vi "Edycja_kursorow_.vi"(7 "Wykres":waveform(dbl)[](array[waveform]), 8 "error in (no error)":errorcluster, 10 "Zablokowane free in":T1[](array[typedef]), 11 "Wykres Ref":refnum<vi>) -> (0 "error out":errorcluster, 2 "Zablokowane free out":T1[](array[typedef]))   [LabVIEW 2013]
uses:
  Kontrolki/GUI/Edycja_blokowanie_free.ctl
panel:
  in  "(Kursor 2)":i32(ring) caption="Lista przebiegów" items=["Przebieg 0", "Przebieg 1", "Przebieg 2", "Przebieg 3", "Kursor", "\"Swobodny\""]
  in  "(Kursor 1)":i32(ring) caption="Lista przebiegów" items=["Przebieg 0", "Przebieg 1", "Przebieg 2", "Przebieg 3", "Kursor", "\"Swobodny\""]
  in  "Lista aktywnych kursorów":i32(ring) items=["Pom1", "Pom2", "Kur_swob", "Kur_2_3"]
  in  "Cancel Button":bool
  in  "OK Button":bool
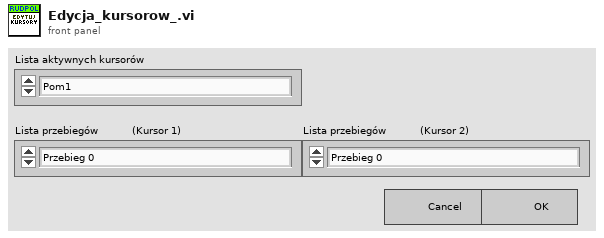
[diagram p1: front panel]
types:
  T1 = typedef "Edycja_blokowanie_free.ctl" = cluster{"Pozycja Y":dbl, "Pozycja X":dbl, "BlokujX":bool, "BlokujY":bool, "Zablokowane":i32}
  T2 = cluster{"Aktywny kursor":i32, "typ kursora":u32, "Aktywne przebiegi":i32[]}
  T3 = typedef "LVCursorListTypeDef.ctl" = cluster{"Name":string, "Color":u32, "Style":u8, "Point Style":u8, "Name Visible":bool, "Allow Drag":bool, "Cursor Mode":u32, "Plot":i32, "Index":i32, "Position":cluster{"X":dbl, "Y":dbl}, "X Scale":u32, "Y Scale":u32, "Watch Plots":i32[], "Watch All Plots":bool, "Plot Area":i32, "Label Offset":cluster{"X":dbl, "Y":dbl}}[]
  T4 = cluster{"Name":string, "Color":u32, "Style":u8, "Point Style":u8, "Name Visible":bool, "Allow Drag":bool, "Cursor Mode":u32, "Plot":i32, "Index":i32, "Position":cluster{"X":dbl, "Y":dbl}, "X Scale":u32, "Y Scale":u32, "Watch Plots":i32[], "Watch All Plots":bool, "Plot Area":i32, "Label Offset":cluster{"X":dbl, "Y":dbl}}
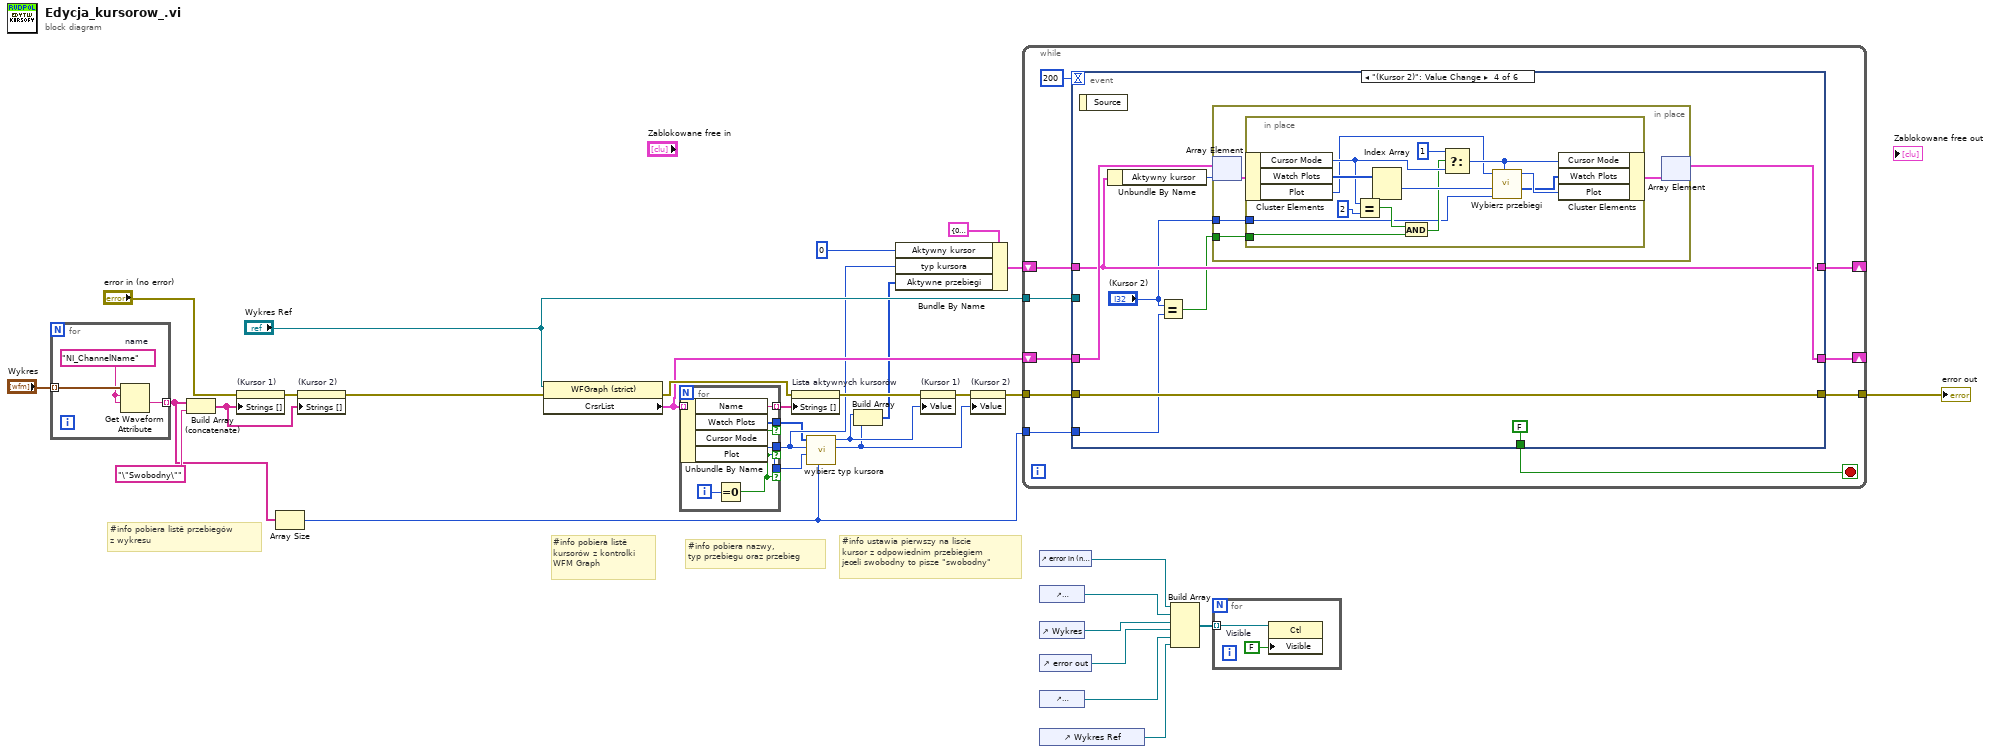
[diagram p0: block diagram]
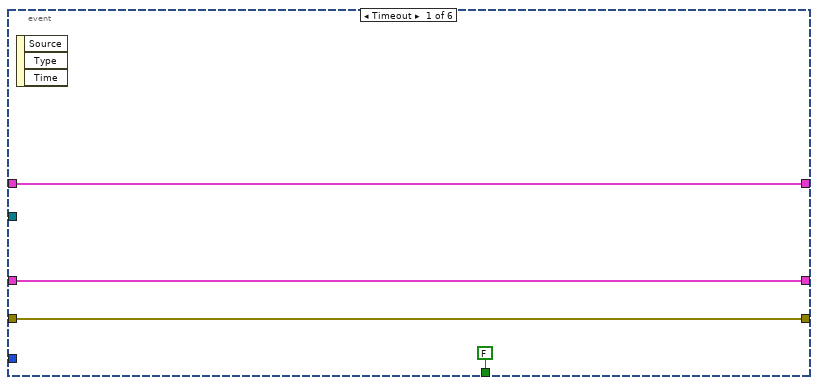
[diagram p2: hidden frame]
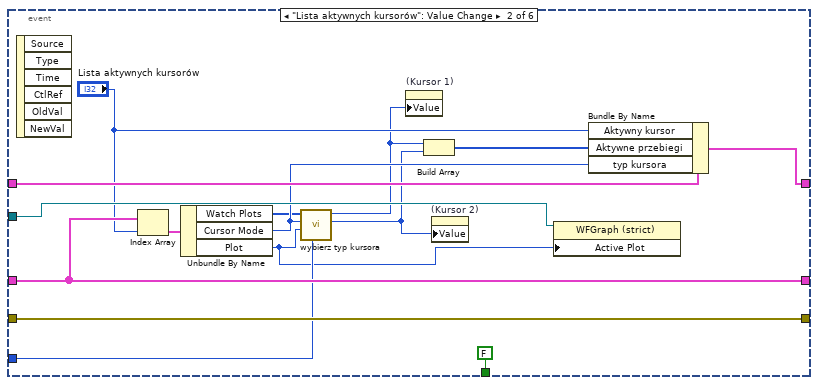
[diagram p3: hidden frame]
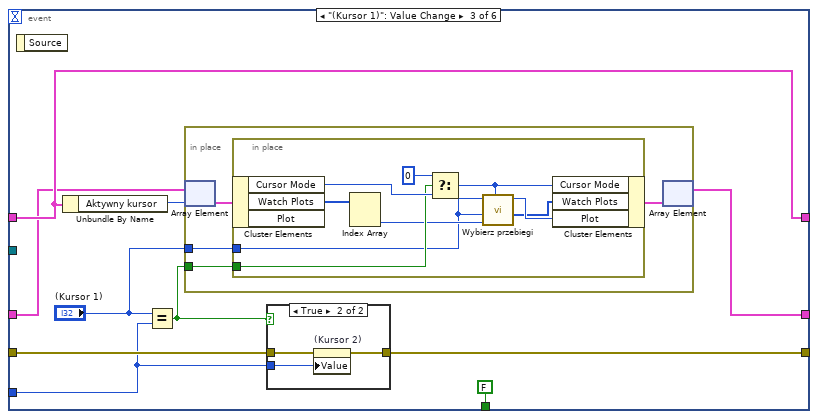
[diagram p4: hidden frame]
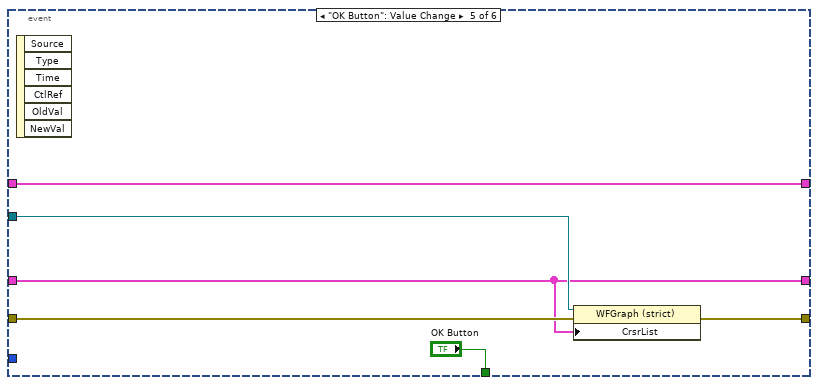
[diagram p6: hidden frame]
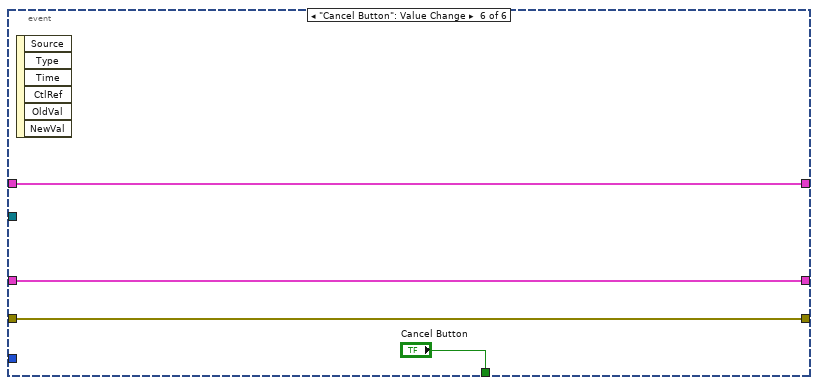
[diagram p7: hidden frame]
diagram:
  # "#info ustawia pierwszy na liscie\nkursor z odpowiednim przebiegiem\njeœli swobodny to pisze \"swobodny\""
  # "#info pobiera nazwy,\ntyp przebiegu oraz przebieg"
  # "#info pobiera listê\nkursorów z kontrolki\nWFM Graph"
  # "#info pobiera listê przebiegów\nz wykresu"
  n1 = for {
    tunnel: "Wykres" -> [w35] mode=indexing
    tunnel: [w33] -> w19 mode=indexing
    w34 = "NI_ChannelName"  # name
    n2 = Get Waveform Attribute(5:w34, 6:w34, 7:w35) -> (1:w33:string)  [unwired: 1 in, 3 out]
  }
  n3 = Build Array (concatenate)(w19, "\"Swobodny\"") -> (w13:string[])
  n4 = property on="(Kursor 1)" class="Ring (strict)"(error in="error in (no error)", "Strings []"=w13) -> (error out=w14:errorcluster)  [unwired: 1 in, 1 out]
  n5 = Array Size(array=w19) -> (size(s)=w11:i32)
  n6 = property on="(Kursor 2)" class="Ring (strict)"(error in=w14, "Strings []"=w13) -> (error out=w10:errorcluster)  [unwired: 1 in, 1 out]
  n7 = property class="WFGraph (strict)"(reference="Wykres Ref", error in=w10) -> (error out=w24:errorcluster, "CrsrList"=w15:T3)  [unwired: 1 out]
  n8 = for {
    tunnel: w15 -> [w42] mode=indexing
    tunnel: [w41] -> w20 mode=indexing
    tunnel: [w40] -> w5 if=w36
    tunnel: [w39] -> w6 if=w36
    tunnel: [w37] -> w4 if=w36
    i -> [w38]
    n9 = Unbundle By Name(w42) -> ("Name"=w41:string, "Watch Plots"=w40:i32[], "Cursor Mode"=w39:u32, "Plot"=w37:i32)
    n10 = Equal To 0?(x=w38) -> (x = 0?=w36:bool)
  }
  n11 = property on="Lista aktywnych kursorów" class="Ring (strict)"(error in=w24, "Strings []"=w20) -> (error out=w8:errorcluster)  [unwired: 1 in, 1 out]
  n12 = call "wybierz typ kursora.vi"("Swobodny"=w11, "Plot in"=w4, "Cursor Mode"=w6, "Plots in"=w5) -> ("Plot2 out"=w2:i32, "Plot1 out"=w3:i32)  [unwired: 6 in]
  n13 = Build Array(w3, w2) -> (w1:i32[])
  n14 = Bundle By Name(cluster=T2 {"Aktywny kursor"=0, "typ kursora"=0, "Aktywne przebiegi"=[]}, "Aktywny kursor"=0, "typ kursora"=w6, "Aktywne przebiegi"=w1) -> (w16:T2)
  n15 = property on="(Kursor 1)" class="Ring (strict)"(error in=w8, "Value"=w3) -> (error out=w7:errorcluster)  [unwired: 1 in, 1 out]
  n16 = property on="(Kursor 2)" class="Ring (strict)"(error in=w7, "Value"=w2) -> (error out=w9:errorcluster)  [unwired: 1 in, 1 out]
  n17 = while {
    tunnel: w9 -> [w52]
    tunnel: [w51] -> w32
    tunnel: "Wykres Ref" -> [w48]
    shift-right: [w46] -> _
    shift-left: w16 -> [w47]
    shift-right: [w44] -> _
    shift-left: w15 -> [w45]
    tunnel: w11 -> [w43]
    stop <- w50 stop-if-true
    n18 = event shown="[3] \"(Kursor 2)\": Value Change" {
      selector: _ -> [_ _ _ _ _ _]
      dyn-events: _ -> [_ _ _ _ _ _]
      timeout: 200 -> [_ _ _ _ _ _]
      tunnel: w52 -> [w55 w70 w75 w107 w128 w134]
      tunnel: [w55 w70 w74 w107 w127 w134] -> w51
      tunnel: [FALSE ("Cancel Button") FALSE ("Cancel Button") FALSE ("Cancel Button") FALSE ("Cancel Button") "OK Button" "Cancel Button"] -> w50
      tunnel: w48 -> [_ w68 _ _ w126 _]
      tunnel: w47 -> [w54 w66 w80 w104 w129 w132]
      tunnel: [w54 w64 w80 w104 w129 w132] -> w46
      tunnel: w45 -> [w53 w67 w79 w106 w125 w131]
      tunnel: [w53 w67 w78 w105 w125 w131] -> w44
      tunnel: w43 -> [_ w63 w72 w101 _ _]
      event Timeout {
        n19 = event-data() -> ()  [unwired: 1 in, 3 out]
      }
      event "Lista aktywnych kursorów": Value Change {
        n20 = event-data() -> ()  [unwired: 1 in, 6 out]
        n21 = Index Array(array=w67, index="Lista aktywnych kursorów") -> (element=w69:T4)
        n22 = Unbundle By Name(w69) -> ("Watch Plots"=w61:i32[], "Cursor Mode"=w62:u32, "Plot"=w60:i32)
        n23 = call "wybierz typ kursora.vi"("Swobodny"=w63, "Plot in"=w60, "Cursor Mode"=w62, "Plots in"=w61) -> ("Plot2 out"=w58:i32, "Plot1 out"=w57:i32)  [unwired: 6 in]
        n24 = property on="(Kursor 1)" class="Ring (strict)"("Value"=w57) -> ()  [unwired: 2 in, 2 out]
        n25 = Build Array(w57, w58) -> (w59:i32[])
        n26 = property on="(Kursor 2)" class="Ring (strict)"("Value"=w58) -> ()  [unwired: 2 in, 2 out]
        n27 = property class="WFGraph (strict)"(reference=w68, "Active Plot"=w60) -> ()  [unwired: 1 in, 2 out]
        n28 = Bundle By Name(cluster=w66, "Aktywny kursor"="Lista aktywnych kursorów", "Aktywne przebiegi"=w59, "typ kursora"=w62) -> (w64:T2)
      }
      event "(Kursor 1)": Value Change {
        n29 = event-data() -> ()  [unwired: 1 in, 1 out]
        n30 = Unbundle By Name(w80) -> ("Aktywny kursor"=w77:i32)
        n31 = Equal?(x="(Kursor 1)", y=w72) -> (x = y?=w73:bool)
        n32 = in-place {
          in-place-border: w73 -> [w87]
          in-place-border: "(Kursor 1)" -> [w86]
          n33 = in-place-array #1(w79, w77) -> (w89:T4)
          n34 = in-place {
            in-place-border: w87 -> [w96]
            in-place-border: w86 -> [w90]
            n35 = in-place-cluster #2(w89) -> ("Cursor Mode"=w98:u32, "Watch Plots"=w93:i32[])  [unwired: 1 out]
            n36 = Index Array(array=w93) -> (element #2=w92:i32)  [unwired: 2 in, 1 out]
            n37 = Select(t=u32 0, s=w96, f=w98) -> (s? t:f=w97:u32)
            n38 = call "Wybierz przebiegi.vi"("Mode"=w97, "Wybierz drugi monitorowanyprzebieg"=w92, "Wybierz pierwszy monitorowanyprzebieg"=w90, "Wybierz monitorowany przebieg"=w90) -> ("WPlots"=w94:i32[], "Plot"=w95:i32)  [unwired: 6 in]
            n39 = in-place-cluster #2("Cursor Mode"=w97, "Watch Plots"=w94, "Plot"=w95) -> (w88:T4)
          }
          n40 = in-place-array #1(w88) -> (w78:T3)  [unwired: 1 out]
        }
        n41 = case shown="True" w73 {
          tunnel: w75 -> [w82 w85]
          tunnel: [w82 w84] -> w74
          tunnel: w72 -> [_ w83]
          frame False {
          }
          frame True {
            n42 = property on="(Kursor 2)" class="Ring (strict)"(error in=w85, "Value"=w83) -> (error out=w84:errorcluster)  [unwired: 1 in, 1 out]
          }
        }
      }
      event "(Kursor 2)": Value Change {
        n43 = event-data() -> ()  [unwired: 1 in, 1 out]
        n44 = Unbundle By Name(w104) -> ("Aktywny kursor"=w103:i32)
        n45 = Equal?(x="(Kursor 2)", y=w101) -> (x = y?=w102:bool)
        n46 = in-place {
          in-place-border: w102 -> [w109]
          in-place-border: "(Kursor 2)" -> [w108]
          n47 = in-place-array #3(w106, w103) -> (w111:T4)
          n48 = in-place {
            in-place-border: w109 -> [w118]
            in-place-border: w108 -> [w112]
            n49 = in-place-cluster #4(w111) -> ("Cursor Mode"=w116:u32, "Watch Plots"=w121:i32[], "Plot"=w113:i32)
            n50 = Equal?(x=w116, y=u32 2 ("x")) -> (x = y?=w117:bool)
            n51 = Index Array(array=w121) -> (element #1=w120:i32)  [unwired: 2 in, 1 out]
            n52 = And(x=w117, y=w118) -> (x .and. y?=w114:bool)
            n53 = Select(t=u32 1, s=w114, f=w116) -> (s? t:f=w124:u32)
            n54 = call "Wybierz przebiegi.vi"("Mode"=w124, "Wybierz drugi monitorowanyprzebieg"=w112, "Wybierz pierwszy monitorowanyprzebieg"=w120, "Wybierz monitorowany przebieg"=w113) -> ("WPlots"=w122:i32[], "Plot"=w123:i32)  [unwired: 6 in]
            n55 = in-place-cluster #4("Cursor Mode"=w124, "Watch Plots"=w122, "Plot"=w123) -> (w110:T4)
          }
          n56 = in-place-array #3(w110) -> (w105:T3)  [unwired: 1 out]
        }
      }
      event "OK Button": Value Change {
        n57 = event-data() -> ()  [unwired: 1 in, 6 out]
        n58 = property class="WFGraph (strict)"(reference=w126, error in=w128, "CrsrList"=w125) -> (error out=w127:errorcluster)  [unwired: 1 out]
      }
      event "Cancel Button": Value Change {
        n59 = event-data() -> ()  [unwired: 1 in, 6 out]
      }
    }
  }
  "error out" <- w32
  n60 = control-ref of="error in (no error)"() -> (w31:refnum<vi>)
  n61 = control-ref of="Zablokowane free in"() -> (w30:refnum<vi>)
  n62 = control-ref of="Wykres"() -> (w29:refnum<vi>)
  n63 = control-ref of="error out"() -> (w27:refnum<vi>)
  n64 = control-ref of="Zablokowane free out"() -> (w26:refnum<vi>)
  n65 = control-ref of="Wykres Ref"() -> (w25:refnum<vi>)
  n66 = Build Array(w31, w30, w29, w27, w26, w25) -> (w28:refnum<vi>[])
  n67 = for {
    tunnel: w28 -> [w136] mode=indexing
    w135 = FALSE  # Visible
    n68 = property class="Ctl"(reference=w136, "Visible"=w135) -> ()  [unwired: 1 in, 2 out]
  }
